vi "Set protocol data.vi"(5 "AK?":bool, 7 "Operation":T1, 8 "error in (no error)":errorcluster, 10 "Localhost Protocols.lvlib:Protocol Parent.lvclass":refnum<class "Protocol Parent.lvclass">, 11 "Listener In.lvclass":refnum<class "Listener.lvclass"> caption="Listener") -> (0 "error out":errorcluster, 3 "Listener Out.lvclass":refnum<class "Listener.lvclass">)   [LabVIEW 2019, in "Listener.lvclass"]
uses:
  Listener.lvclass
  ListenerClassControls/Operation Ctl.ctl
  Protocol Parent/Protocol Parent.lvclass
  ListenerClassControls/TCP IP Data Structure.ctl
  TCP/TCP.lvclass
  TCP/TCP.lvclass/TCP.ctl
  AK TCP/AK TCP.lvclass
  D:/GitRepository/niveristand-instrument-addon-classes/Source/Protocols/TCP/TCP.lvclass
  ListenerClassControls/AK TCP IP Data Structure.ctl
  UDP/UDP.lvclass
  ListenerClassControls/UDP Data Structure.ctl
  UDP/UDP.lvclass/UDP.ctl
  TCP/Data Access/Read IP Address.vi
  TCP/Data Access/Read Port.vi
  UDP/Data Access/Read Target IP Address.vi
  UDP/Data Access/Read Local Port.vi
  UDP/Data Access/Read Local IP Address.vi
  UDP/Data Access/Read Target Port.vi
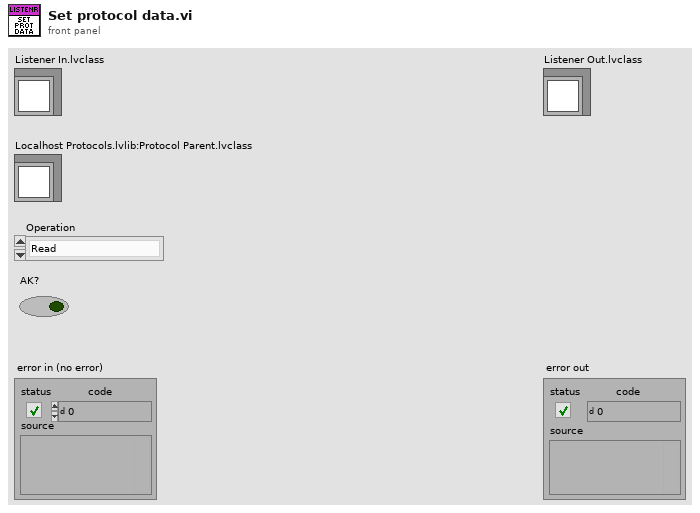
[diagram p1: front panel]
types:
  T1 = typedef "Operation Ctl.ctl" = enum16{"Read", "Write"}
  T2 = typedef "Listener.lvclass/TCP IP Data Structure.ctl" = cluster{"TCP|IP connection ID":refnum<k5>, "IP Address":string, "Port":u16, "Data":string}
  T3 = typedef "Listener.lvclass/AK TCP IP Data Structure.ctl" = cluster{"TCP|IP connection ID":refnum<k5>, "IP Address":string, "Port":u16, "Data":string, "Current Command Code":string}
  T4 = typedef "Listener.lvclass/UDP Data Structure.ctl" = cluster{"UDP connection ID":refnum<k16>, "Local Address":string, "Local Port":u16, "Target IP Address":string, "Target Port":u16, "Data":string}
  T5 = typedef "Localhost Protocols.lvlib/Protocol Parent.lvclass/Base Protocol Type.ctl" = enum16{"RS-XXX", "VISA", "TCPIP", "UDP", "GPIB ConvBox"}
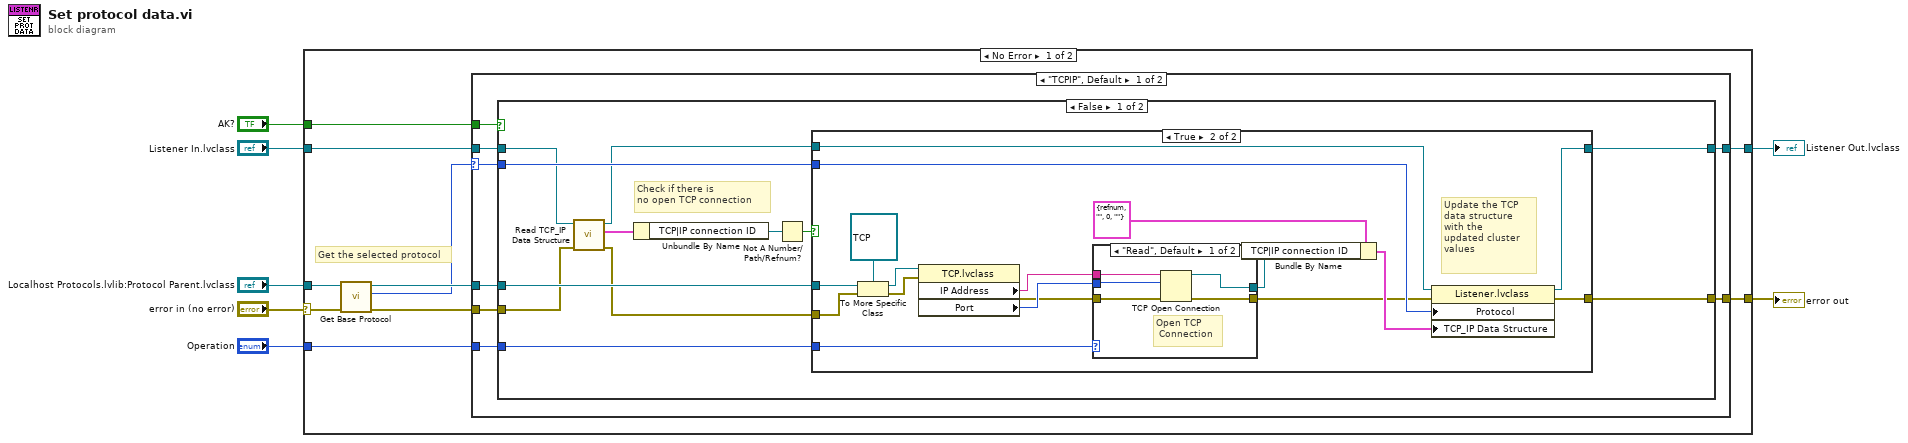
[diagram p0: block diagram]
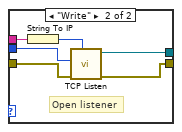
[diagram p3: hidden frame]
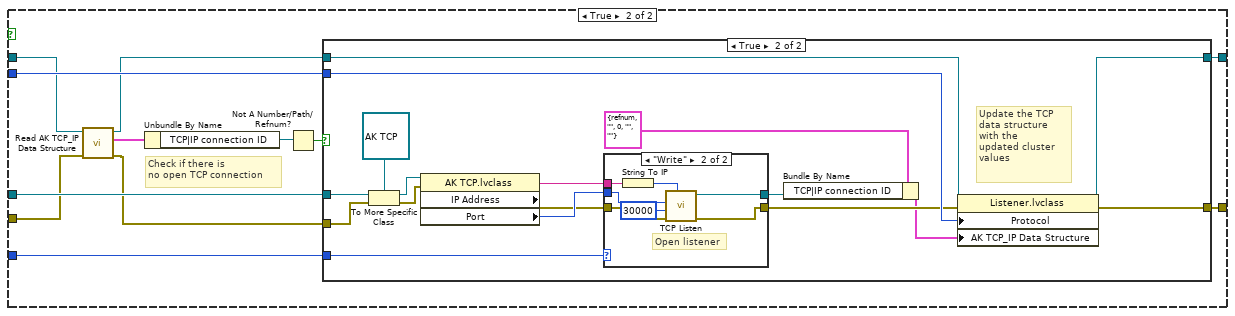
[diagram p4: hidden frame]
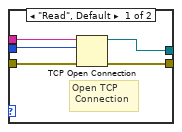
[diagram p6: hidden frame]
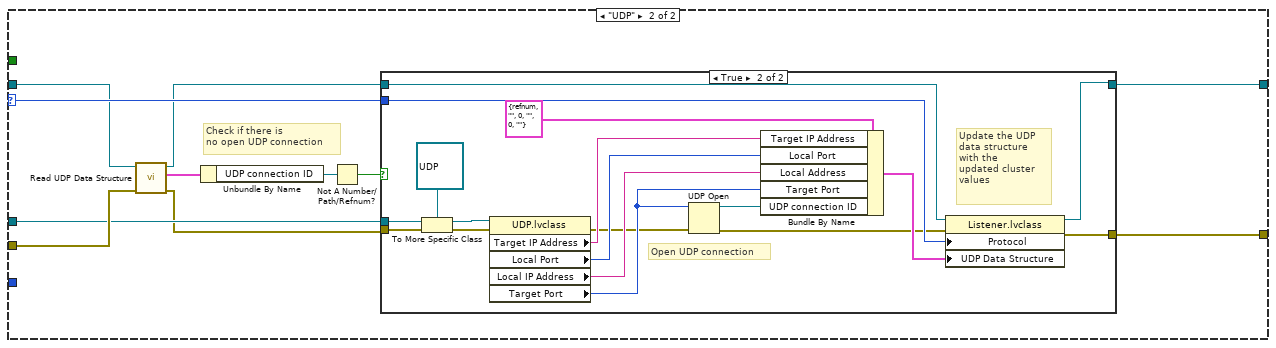
[diagram p7: hidden frame]
diagram:
  n1 = case shown="No Error" "error in (no error)" {
    selector: "error in (no error)" -> [w11 w143]
    tunnel: [w17 w143] -> w6
    tunnel: "Localhost Protocols.lvlib:Protocol Parent.lvclass" -> [w12 _]
    tunnel: "Listener In.lvclass" -> [w16 w142]
    tunnel: [w15 w142] -> w4
    tunnel: "Operation" -> [w14 _]
    tunnel: "AK?" -> [w13 _]
    frame No Error {
      # "Get the selected protocol"
      n2 = call-dynamic "Get Base Protocol.vi"("error in (no error)"=w11, "Protocol Parent in"=w12) -> ("error out"=w10:errorcluster, "Protocol out"=w8:T5, "Protocol Parent out"=w9:refnum<class "Protocol Parent.lvclass">)  [unwired: 7 in]
      n3 = case shown="\"TCPIP\", Default" w8 {
        selector: w8 -> [w23 w120]
        tunnel: w9 -> [w25 w114]
        tunnel: w10 -> [w20 w116]
        tunnel: [w22 w119] -> w17
        tunnel: w16 -> [w21 w115]
        tunnel: [w24 w121] -> w15
        tunnel: w14 -> [w19 _]
        tunnel: w13 -> [w18 _]
        frame "TCPIP", Default {
          n4 = case shown="False" w18 {
            tunnel: w25 -> [w37 w79]
            tunnel: [w36 w78] -> w24
            tunnel: w23 -> [w35 w77]
            tunnel: [w34 w76] -> w22
            tunnel: w21 -> [w32 w73]
            tunnel: w20 -> [w31 w71]
            tunnel: w19 -> [w26 w74]
            frame False {
              # "Check if there is \nno open TCP connection"
              n5 = call-dynamic "Read TCP_IP Data Structure.vi"("error in (no error)"=w31, "Listener in"=w32) -> ("error out"=w30:errorcluster, "TCP|IP Data Structure"=w29:T2, "Listener out"=w28:refnum<class "Listener.lvclass">)  [unwired: 7 in]
              n6 = Unbundle By Name(w29) -> ("TCP|IP connection ID"=w33:refnum<k5>)
              n7 = Not A Number/Path/Refnum?(number/path/refnum=w33) -> (NaN/Path/Refnum?=w27:bool)
              n8 = case shown="True" w27 {
                tunnel: w37 -> [_ w56]
                tunnel: [w39 w52] -> w36
                tunnel: w35 -> [_ w51]
                tunnel: [w38 w49] -> w34
                tunnel: w30 -> [w38 w48]
                tunnel: w28 -> [w39 w47]
                tunnel: w26 -> [_ w46]
                frame False {
                }
                frame True {
                  # "Update the TCP \ndata structure\nwith the\nupdated cluster\nvalues"
                  n9 = To More Specific Class(target class=refnum<class "TCP.lvclass"> refnum ("Localhost Protocols.lvlib:TCP.lvclass"), reference=w56, error in=w48) -> (specific class reference=w55:refnum<class "TCP.lvclass">, error out=w54:errorcluster)
                  n10 = property class="TCP.lvclass"(reference=w55, error in=w54) -> (error out=w44:errorcluster, "IP Address"=w43:string, "Port"=w45:u16)  [unwired: 1 out]
                  n11 = case shown="\"Read\", Default" w46 {
                    tunnel: w45 -> [w61 w66]
                    tunnel: w44 -> [w60 w67]
                    tunnel: w43 -> [w59 w65]
                    tunnel: [w58 w62] -> w42
                    tunnel: [w57 w63] -> w41
                    frame "Read", Default {
                      # "Open TCP\n Connection"
                      n12 = TCP Open Connection(address=w59, remote port or service name=w61, error in (no error)=w60) -> (connection ID=w57:refnum<k5>, error out=w58:errorcluster)  [unwired: 2 in]
                    }
                    frame "Write" {
                      # "Open listener"
                      n13 = String To IP(1:w65) -> (0:w64:u32)
                      n14 = call <vilib>:"TCP Listen.vi"("net address"=w64, "error in (no error)"=w67, "port"=w66) -> ("error out"=w62:errorcluster, "connection ID"=w63:refnum<k5>)  [unwired: 4 in, 3 out]
                    }
                  }
                  n15 = Bundle By Name(cluster=T2 {"TCP|IP connection ID"=refnum, "IP Address"="", "Port"=0, "Data"=""} ("TCP|IP Data Structure"), "TCP|IP connection ID"=w41) -> (w50:T2)
                  n16 = property class="Listener.lvclass"(reference=w47, error in=w42, "Protocol"=w51, "TCP_IP Data Structure"=w50) -> (reference out=w52:refnum<class "Listener.lvclass">, error out=w49:errorcluster)
                }
              }
            }
            frame True {
              # "Check if there is \nno open TCP connection"
              n17 = call-dynamic "Read AK TCP_IP Data Structure.vi"("error in (no error)"=w71, "Listener in"=w73) -> ("error out"=w70:errorcluster, "TCP|IP Data Structure"=w69:T3, "Listener out"=w72:refnum<class "Listener.lvclass">)  [unwired: 7 in]
              n18 = Unbundle By Name(w69) -> ("TCP|IP connection ID"=w68:refnum<k5>)
              n19 = Not A Number/Path/Refnum?(number/path/refnum=w68) -> (NaN/Path/Refnum?=w75:bool)
              n20 = case shown="True" w75 {
                tunnel: w79 -> [_ w98]
                tunnel: [w81 w95] -> w78
                tunnel: w77 -> [_ w94]
                tunnel: [w80 w93] -> w76
                tunnel: w70 -> [w80 w92]
                tunnel: w72 -> [w81 w91]
                tunnel: w74 -> [_ w90]
                frame False {
                }
                frame True {
                  # "Update the TCP \ndata structure\nwith the\nupdated cluster\nvalues"
                  n21 = To More Specific Class(target class=refnum<class "AK TCP.lvclass"> refnum ("Protocols.lvlib:AK TCP.lvclass"), reference=w98, error in=w92) -> (specific class reference=w97:refnum<class "AK TCP.lvclass">, error out=w96:errorcluster)
                  n22 = property class="AK TCP.lvclass"(reference=w97, error in=w96) -> (error out=w88:errorcluster, "IP Address"=w87:string, "Port"=w89:u16)  [unwired: 1 out]
                  n23 = case shown="\"Write\"" w90 {
                    tunnel: w89 -> [w103 w105]
                    tunnel: w88 -> [w102 w110]
                    tunnel: w87 -> [w101 w109]
                    tunnel: [w100 w106] -> w86
                    tunnel: [w99 w107] -> w85
                    frame "Read", Default {
                      # "Open TCP\n Connection"
                      n24 = TCP Open Connection(address=w101, remote port or service name=w103, error in (no error)=w102) -> (connection ID=w99:refnum<k5>, error out=w100:errorcluster)  [unwired: 2 in]
                    }
                    frame "Write" {
                      # "Open listener"
                      n25 = String To IP(1:w109) -> (0:w108:u32)
                      n26 = call <vilib>:"TCP Listen.vi"("net address"=w108, "error in (no error)"=w110, "timeout ms (wait forever: -1)"=30000, "port"=w105) -> ("error out"=w106:errorcluster, "connection ID"=w107:refnum<k5>)  [unwired: 3 in, 3 out]
                    }
                  }
                  n27 = Bundle By Name(cluster=T3 {"TCP|IP connection ID"=refnum, "IP Address"="", "Port"=0, "Data"="", "Current Command Code"=""} ("TCP|IP Data Structure"), "TCP|IP connection ID"=w85) -> (w82:T3)
                  n28 = property class="Listener.lvclass"(reference=w91, error in=w86, "Protocol"=w94, "AK TCP_IP Data Structure"=w82) -> (reference out=w95:refnum<class "Listener.lvclass">, error out=w93:errorcluster)
                }
              }
            }
          }
        }
        frame "UDP" {
          # "Check if there is \nno open UDP connection"
          n29 = call-dynamic "Read UDP Data Structure.vi"("error in (no error)"=w116, "Listener in"=w115) -> ("error out"=w112:errorcluster, "UDP Data Structure"=w113:T4, "Listener out"=w111:refnum<class "Listener.lvclass">)  [unwired: 7 in]
          n30 = Unbundle By Name(w113) -> ("UDP connection ID"=w117:refnum<k16>)
          n31 = Not A Number/Path/Refnum?(number/path/refnum=w117) -> (NaN/Path/Refnum?=w118:bool)
          n32 = case shown="True" w118 {
            tunnel: w112 -> [w123 w141]
            tunnel: w114 -> [_ w139]
            tunnel: w111 -> [w122 w133]
            tunnel: [w122 w132] -> w121
            tunnel: w120 -> [_ w130]
            tunnel: [w123 w129] -> w119
            frame False {
            }
            frame True {
              # "Update the UDP \ndata structure\nwith the\nupdated cluster\nvalues"
              # "Open UDP connection"
              n33 = To More Specific Class(target class=refnum<class "UDP.lvclass"> refnum ("Protocols.lvlib:UDP.lvclass"), reference=w139, error in=w141) -> (specific class reference=w128:refnum<class "UDP.lvclass">, error out=w138:errorcluster)
              n34 = property class="UDP.lvclass"(reference=w128, error in=w138) -> (error out=w126:errorcluster, "Target IP Address"=w137:string, "Local Port"=w136:u16, "Local IP Address"=w135:string, "Target Port"=w127:u16)  [unwired: 1 out]
              n35 = UDP Open(8:w126, 11:w127) -> (port=w125:refnum<k16>, 0:w124:errorcluster)  [unwired: 3 in, 1 out]
              n36 = Bundle By Name(cluster=T4 {"UDP connection ID"=refnum, "Local Address"="", "Local Port"=0, "Target IP Address"="", "Target Port"=0, "Data"=""} ("UDP Data Structure"), "Target IP Address"=w137, "Local Port"=w136, "Local Address"=w135, "Target Port"=w127, "UDP connection ID"=w125) -> (w131:T4)
              n37 = property class="Listener.lvclass"(reference=w133, error in=w124, "Protocol"=w130, "UDP Data Structure"=w131) -> (reference out=w132:refnum<class "Listener.lvclass">, error out=w129:errorcluster)
            }
          }
        }
      }
    }
    frame Error {
    }
  }
  "Listener Out.lvclass" <- w4
  "error out" <- w6
